vi "CleanViName.vi"(11 "Name":string) -> (3 "submatch 1":string)   [LabVIEW 2017]
uses:
  <vilib>/regexp/Match Regular Expression.xnode
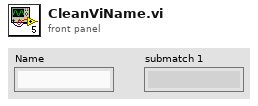
[diagram p1: front panel]
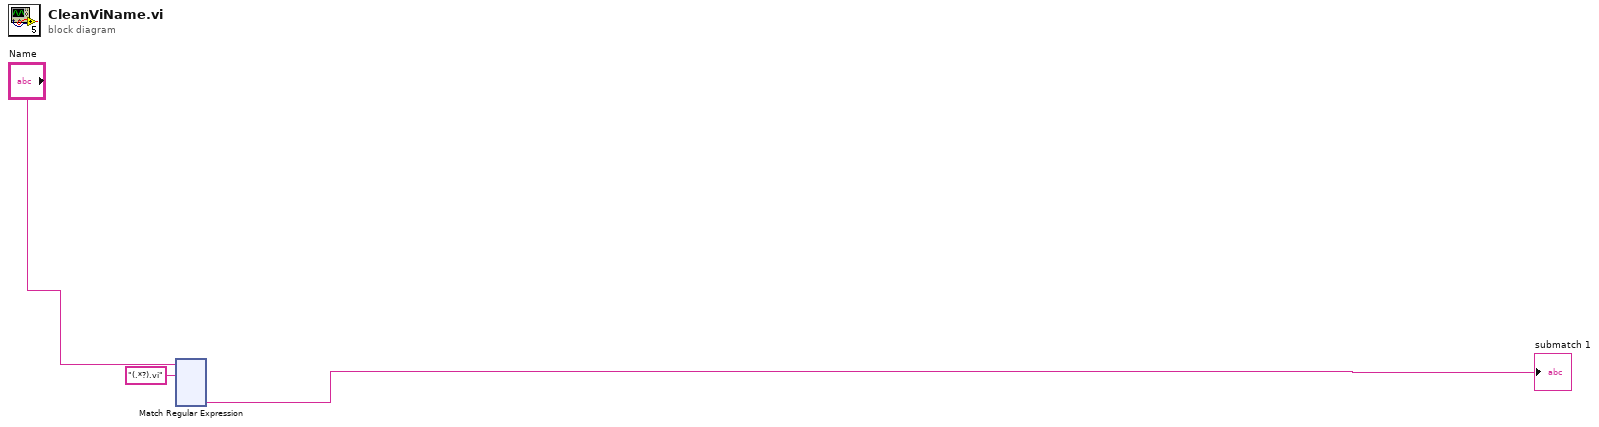
[diagram p0: block diagram]
diagram:
  n1 = xnode "Match Regular Expression"("input string"="Name", "regular expression"="(.*?).vi") -> ("submatch 1"=→"submatch 1":string)  [unwired: 4 in, 5 out]
